vi "createState.vi"(8 "error in (no error)":errorcluster, 10 "stateValue":T1, 11 "StateFactory in":refnum<class "StateFactory.lvclass">) -> (0 "error out":errorcluster, 2 "state":refnum<class "State.lvclass">, 3 "StateFactory out":refnum<class "StateFactory.lvclass">)   [LabVIEW 2016, in "StateFactory.lvclass"]
uses:
  StateFactory.lvclass
  Typedefs/StateValue.ctl
  State/State.lvclass
  States/DisabledState/DisabledState.lvclass
  home/andres/ct_cmpuserevents/States/DefaultState/DefaultState.lvclass
  States/EnabledState/EnabledState.lvclass
  States/FaultState/FaultState.lvclass
  States/OffState/OffState.lvclass
  States/StandbyState/StandbyState.lvclass
  States/DefaultState/DefaultState.lvclass
  home/andres/ct_cmpuserevents/State/State.lvclass
  Typedefs/EXATypedefs.lvlib
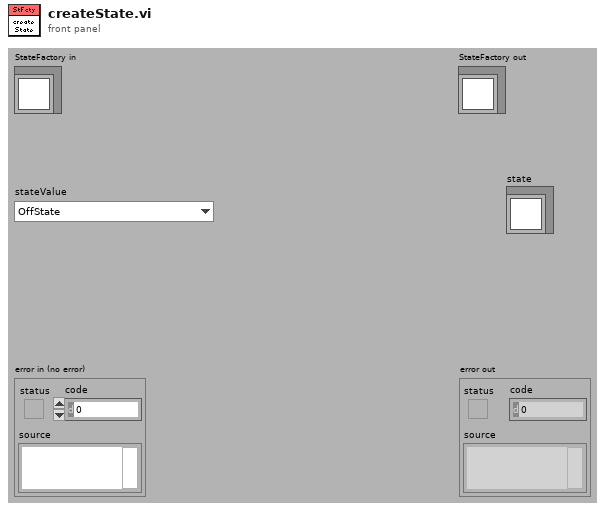
[diagram p1: front panel]
types:
  T1 = typedef "EXATypedefs.lvlib/StateValue.ctl" = enum16{"OffState", "StandbyState", "DisabledState", "EnabledState", "FaultState"}
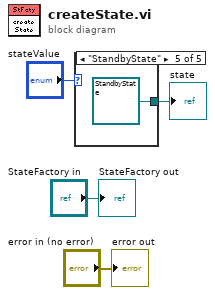
[diagram p0: block diagram]
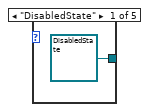
[diagram p2: hidden frame]
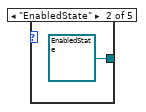
[diagram p3: hidden frame]
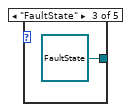
[diagram p4: hidden frame]
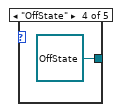
[diagram p5: hidden frame]
diagram:
  n1 = case shown="\"StandbyState\"" "stateValue" {
    tunnel: [refnum<class "DisabledState.lvclass"> refnum ("DisabledState.lvclass") refnum<class "EnabledState.lvclass"> refnum ("States.lvlib:EnabledState.lvclass") refnum<class "FaultState.lvclass"> refnum ("FaultState.lvclass") refnum<class "OffState.lvclass"> refnum ("OffState.lvclass") refnum<class "StandbyState.lvclass"> refnum ("StandbyState.lvclass")] -> w4
    frame "DisabledState" {
    }
    frame "EnabledState" {
    }
    frame "FaultState" {
    }
    frame "OffState" {
    }
    frame "StandbyState" {
    }
  }
  "state" <- w4
  "error out" <- "error in (no error)"
  "StateFactory out" <- "StateFactory in"
